vi "current_ramp_FSM.vi"(0 "commands":refnum<queue>, 2 "State":refnum<queue>) -> ()   [LabVIEW 2021]
uses:
  <vilib>/ErrorRing/Error Ring.xnode
panel:
  out "State":string
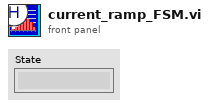
[diagram p1: front panel]
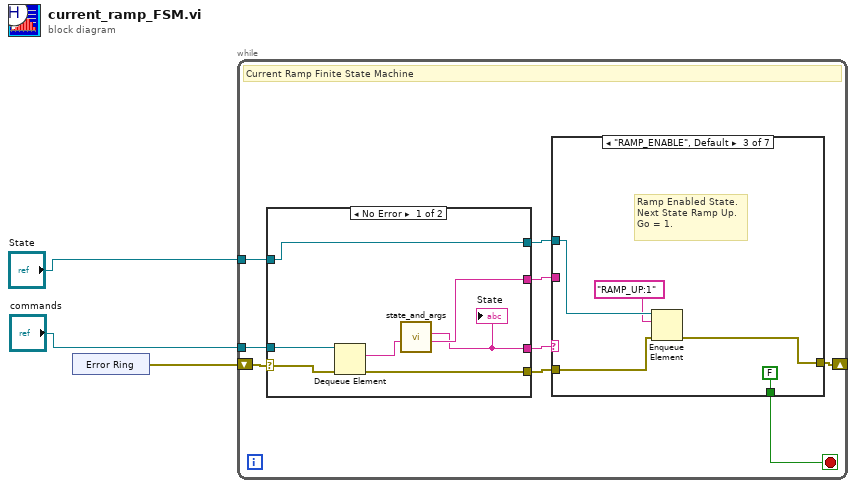
[diagram p0: block diagram]
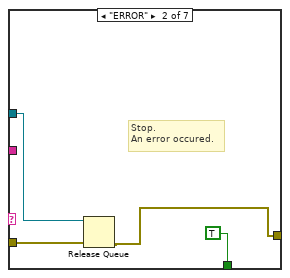
[diagram p3: hidden frame]
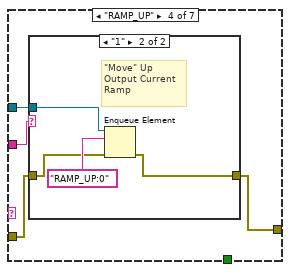
[diagram p4: hidden frame]
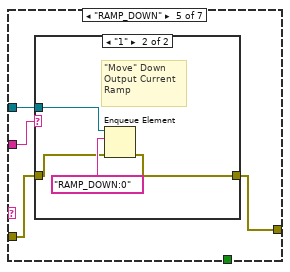
[diagram p6: hidden frame]
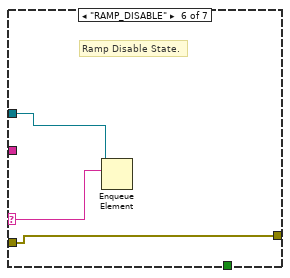
[diagram p8: hidden frame]
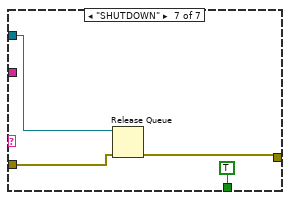
[diagram p9: hidden frame]
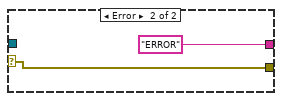
[diagram p10: hidden frame]
diagram:
  n1 = xnode "Error Ring"() -> ("error out"=w3:errorcluster)
  n2 = while {
    shift-right: [w11] -> _
    shift-left: w3 -> [w12]
    tunnel: "commands" -> [w7]
    tunnel: "State" -> [w4]
    stop <- w6 stop-if-true
    # "Current Ramp Finite State Machine"
    n3 = case shown="No Error" w12 {
      selector: w12 -> [w54 w55]
      tunnel: [w53 w55] -> w10
      tunnel: [w48 "ERROR" ("State")] -> w9
      tunnel: [w52 _] -> w8
      tunnel: w7 -> [w50 _]
      tunnel: [w49 _] -> w5
      tunnel: w4 -> [w49 _]
      frame No Error {
        n4 = Dequeue Element(queue=w50, error in (no error)=w54) -> (element=w51:string, error out=w53:errorcluster)  [unwired: 1 in, 2 out]
        n5 = call "state_and_args.vi"("String"=w51) -> ("Arguments"=w52:string, "State"=w48:string)  [unwired: 9 in]
        "State" <- w48
      }
      frame Error {
      }
    }
    n6 = case shown="\"RAMP_ENABLE\", Default" w9 {
      selector: w9 -> [_ _ _ _ _ w41 _]
      tunnel: [w13 w14 w19 w24 w33 w43 w45] -> w11
      tunnel: w10 -> [w13 w15 w20 w25 w34 w43 w46]
      tunnel: w8 -> [_ _ _ w26 w35 _ _]
      tunnel: [_ TRUE FALSE _ _ _ TRUE] -> w6
      tunnel: w5 -> [_ w16 w21 w23 w32 w42 w47]
      frame "IDLE" {
        # "WAIT."
      }
      frame "ERROR" {
        # "Stop. \nAn error occured."
        n7 = Release Queue(queue=w16, error in (no error)=w15) -> (error out=w14:errorcluster)  [unwired: 1 in, 2 out]
      }
      frame "RAMP_ENABLE", Default {
        # "Ramp Enabled State.\nNext State Ramp Up.\nGo = 1."
        n8 = Enqueue Element(queue=w21, element="RAMP_UP:1", error in (no error)=w20) -> (error out=w19:errorcluster)  [unwired: 1 in, 2 out]
      }
      frame "RAMP_UP" {
        n9 = case shown="\"1\"" w26 {
          tunnel: [w27 w28] -> w24
          tunnel: w25 -> [w27 w29]
          tunnel: w23 -> [_ w31]
          frame "0", Default {
            # "Until the\nNext Value\nis requested\ndon't \"move\"."
          }
          frame "1" {
            # "\"Move\" Up\nOutput Current\nRamp"
            n10 = Enqueue Element(queue=w31, element="RAMP_UP:0", error in (no error)=w29) -> (error out=w28:errorcluster)  [unwired: 1 in, 2 out]
          }
        }
      }
      frame "RAMP_DOWN" {
        n11 = case shown="\"1\"" w35 {
          tunnel: [w36 w37] -> w33
          tunnel: w34 -> [w36 w38]
          tunnel: w32 -> [_ w40]
          frame "0", Default {
            # "Until the\nNext Value\nis requested\ndon't \"move\"."
          }
          frame "1" {
            # "\"Move\" Down\nOutput Current\nRamp"
            n12 = Enqueue Element(queue=w40, element="RAMP_DOWN:0", error in (no error)=w38) -> (error out=w37:errorcluster)  [unwired: 1 in, 2 out]
          }
        }
      }
      frame "RAMP_DISABLE" {
        # "Ramp Disable State."
        n13 = Enqueue Element(queue=w42, element=w41) -> ()  [unwired: 2 in, 3 out]
      }
      frame "SHUTDOWN" {
        n14 = Release Queue(queue=w47, error in (no error)=w46) -> (error out=w45:errorcluster)  [unwired: 1 in, 2 out]
      }
    }
  }
